vi "Create Manager.Text.vi"(5 "ConfigManager.Text":refnum<class "ConfigManager.Text.lvclass">, 6 "read-only?":bool, 8 "error in (no error)":errorcluster, 11 "filepath":path) -> (0 "error out":errorcluster, 2 "CfgManager.Text Public Events":T1, 3 "ConfigManager.Text out":refnum<class "ConfigManager.Text.lvclass">)   [LabVIEW 2013, in "CfgManager.Text.lvlib" / "ConfigManager.Text.lvclass"]
uses:
  ConfigManager.Text.lvclass
  PublicEvents -- Cluster.ctl
  ConfigManager.Text.lvclass/ConfigManager.Text.ctl
  payload -- cluster.ctl
  Response - cluster.ctl
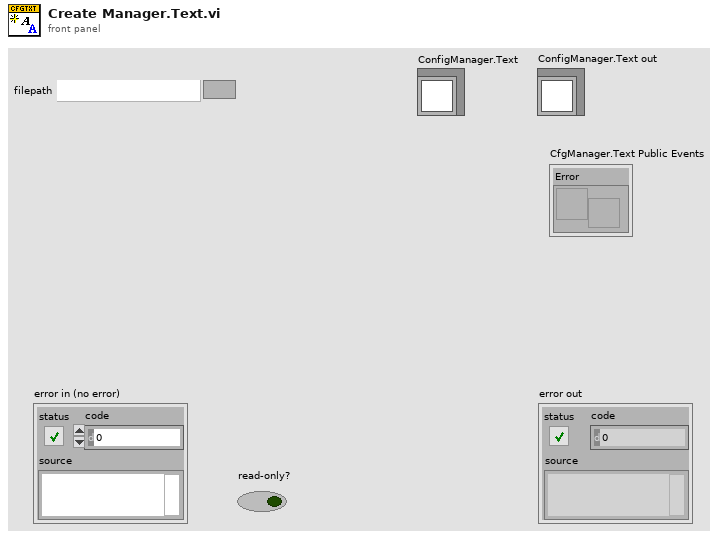
[diagram p1: front panel]
types:
  T1 = typedef "CfgManager.Text.lvlib/ConfigManager.Text.lvclass/PublicEvents -- Cluster.ctl" = cluster{"Error":refnum<user-event>}
  T2 = typedef "CfgManager.Text.lvlib/ConfigManager.Text.lvclass/payload -- cluster.ctl" = cluster{"command":string, "args":variant, "query":refnum<notifier>, "ack":refnum<notifier>}
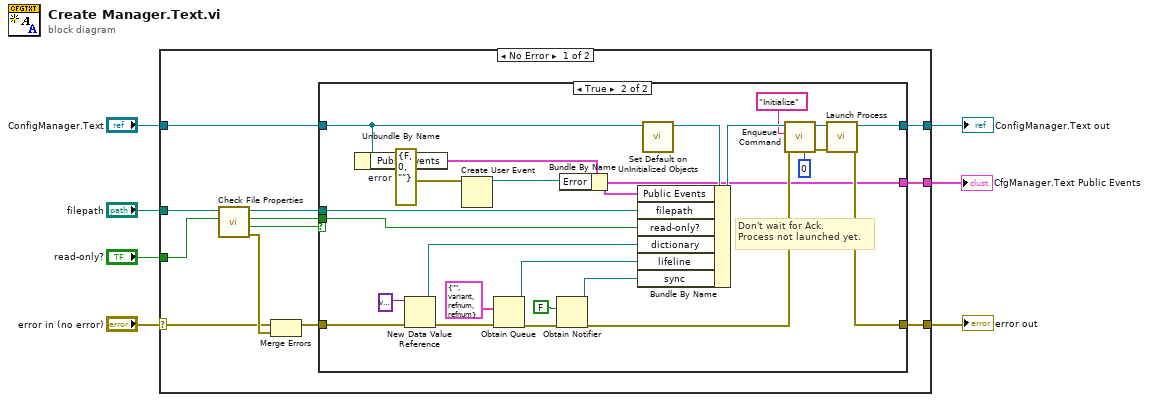
[diagram p0: block diagram]
diagram:
  n1 = case shown="No Error" "error in (no error)" {
    selector: "error in (no error)" -> [w10 w47]
    tunnel: "ConfigManager.Text" -> [w18 w48]
    tunnel: [w17 w48] -> w6
    tunnel: "filepath" -> [w16 _]
    tunnel: [w19 w47] -> w3
    tunnel: "read-only?" -> [w14 _]
    tunnel: [w8 _] -> w1
    frame No Error {
      n2 = call "Check File Properties.vi"("Read-Only?"=w14, "filepath"=w16) -> ("error out"=w11:errorcluster, "File exists"=w12:bool, "Read-Only"=w13:bool, "filepath dup"=w15:path)  [unwired: 5 in, 1 out]
      n3 = Merge Errors(w10, w11) -> (w9:errorcluster)
      n4 = case shown="True" w12 {
        tunnel: [w20 w43] -> w19
        tunnel: w18 -> [w21 w26]
        tunnel: [w21 w41] -> w17
        tunnel: w9 -> [w20 w31]
        tunnel: w15 -> [_ w28]
        tunnel: w13 -> [_ w27]
        tunnel: [_ w22] -> w8
        frame False {
        }
        frame True {
          w24 = errorcluster {"status"=FALSE, "code"=0, "source"=""}  # error
          # "Don't wait for Ack.\nProcess not launched yet."
          n5 = Unbundle By Name(w26) -> ("Public Events"=w23:T1)
          n6 = New Data Value Reference(data value=variant ("Variant"), error in=w31) -> (data value reference=w45:refnum<data-value>, error out=w30:errorcluster)
          n7 = Create User Event(user event datatype=w24) -> (user event=w25:refnum<user-event>)  [unwired: 1 in, 1 out]
          n8 = Obtain Queue(element data type=T2 {"command"="", "args"=variant, "query"=refnum, "ack"=refnum} ("payload"), error in (no error)=w30) -> (queue out=w35:refnum<queue>, error out=w33:errorcluster)  [unwired: 3 in, 1 out]
          n9 = Obtain Notifier(notification data type=FALSE, error in (no error)=w33) -> (notifier out=w34:refnum<notifier>, error out=w32:errorcluster)  [unwired: 2 in, 1 out]
          n10 = Bundle By Name(cluster=w23, "Error"=w25) -> (w22:T1)
          n11 = call "Set Default on UnInitialized Objects.vi"("ConfigManager.Text in"=w26) -> ("ConfigManager.Text out"=w29:refnum<class "ConfigManager.Text.lvclass">)  [unwired: 10 in]
          n12 = Bundle By Name(cluster=w29, "Public Events"=w22, "filepath"=w28, "read-only?"=w27, "dictionary"=w45, "lifeline"=w35, "sync"=w34) -> (w40:refnum<class "ConfigManager.Text.lvclass">)
          n13 = call "Enqueue Command.vi"("ack timeout (0 ms: no ack)"=0 ("ack timeout (ms)"), "error in (no error)"=w32, "command"="Initialize", "ConfigManager.Text in"=w40) -> ("error out"=w36:errorcluster, "ConfigManager.Text out"=w39:refnum<class "ConfigManager.Text.lvclass">)  [unwired: 5 in, 1 out]
          n14 = call-dynamic "Launch Process.vi"("error in (no error)"=w36, "ConfigManager.Text in"=w39) -> ("error out"=w43:errorcluster, "ConfigManager.Text out"=w41:refnum<class "ConfigManager.Text.lvclass">)  [unwired: 7 in, 1 out]
        }
      }
    }
    frame Error {
    }
  }
  "ConfigManager.Text out" <- w6
  "error out" <- w3
  "CfgManager.Text Public Events" <- w1
